vi "getSweepWaveforms.vi"(8 "error in (no error)":errorcluster, 11 "Instrument.LockinAPI in":refnum<class "Instrument.LockinAPI.lvclass">) -> (0 "error out":errorcluster, 1 "Sweep_AI":waveform(dbl)[](array[waveform]), 2 "Sweep_AO":waveform(dbl)[](array[waveform]), 3 "Instrument.LockinAPI out":refnum<class "Instrument.LockinAPI.lvclass">)   [LabVIEW 2019, in "Instrument.LockinAPI.lvclass"]
doc: "API to get the results of lockin calculation.\n\nIf address=\"\", this API reads from localhost\nIf address is remote lockin, you need to add this computer to allowed whitelist on the lockin computer you are trying to access."
uses:
  Instrument.LockinAPI.lvclass
  C:/Users/patrick/Documents/GitHub/Instrument-Framework/lvsrc/Instrument/Instrument.lvclass
  Typedefs/API/LockinAPI.Commands--Enum.ctl
  06e2ff75-1166-4892-8dfd-d8385005f928.vi
  06e2ff75-1166-4892-8dfd-d8385005f928.vi/f68ae031-2bc9-4b14-8172-68b8d1320710.vi
  06e2ff75-1166-4892-8dfd-d8385005f928.vi/f68ae031-2bc9-4b14-8172-68b8d1320710.vi/c120edc0-3eca-4408-adb5-28e9c0c7fff1.vi
  06e2ff75-1166-4892-8dfd-d8385005f928.vi/f68ae031-2bc9-4b14-8172-68b8d1320710.vi/c120edc0-3eca-4408-adb5-28e9c0c7fff1.vi/e50917fa-9e4a-4e04-9c38-a1a604490af2.vi
  06e2ff75-1166-4892-8dfd-d8385005f928.vi/f68ae031-2bc9-4b14-8172-68b8d1320710.vi/c120edc0-3eca-4408-adb5-28e9c0c7fff1.vi/56e2ec84-47dc-4db2-833f-128f254202da.vi
  Instrument/Protected/Validate API method.vi
  Instrument/Private/Get RC Connection Status.vi
  Instrument/API/Send and Receive.vi
  <vilib>/Utility/Data Type/Get Type Information.vi
  <vilib>/JDP Science/JSONtext/JSON text to Variant.vi
  <vilib>/JDP Science/JSONtext/LVClass Serializer/JSONtext LVClass Serializer.lvclass
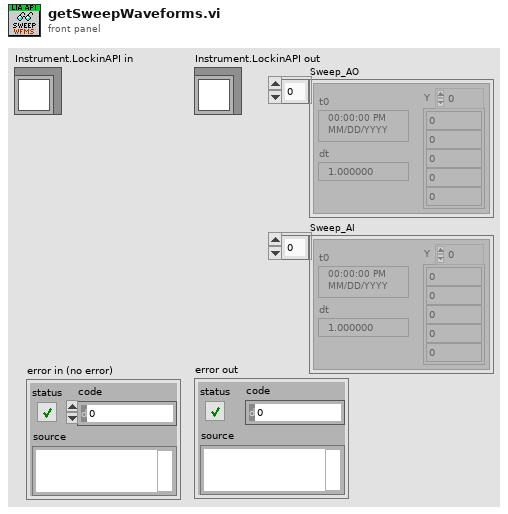
[diagram p1: front panel]
types:
  T1 = typedef "Instrument.LockinAPI.lvclass/LockinAPI.Commands--Enum.ctl" = enum16{"setAI", "setAO", "setAO_Amplitude", "setAO_DC", "setAO_Frequency", "setAO_Phase", "setAO_Function", "setAO_I+", "setREF", "setREF_Frequency", "setREF_Phase", "setREF_TC", "setREF_Roll-Off", "setDAQ", "setSampling", "setOffset", "setState", "getState", "getAO", "getAI", "getResults", "getSampling", "getAOconfig", "getREFconfig", "setInputGain", "setOutputGain", "getInputGain", "getOutputGain", "setSamplingMode", "getSamplingMode", "setSweep", "setSweepTime", "setSweepTable", "getStatus", "getSweepResults", "getSweepWaveforms", "startSweep", "stopSweep", "setAUX", "getAUX"}
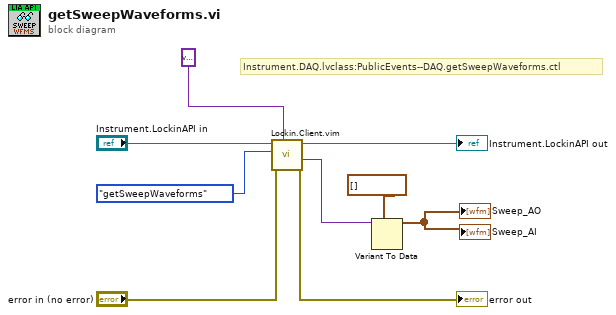
[diagram p0: block diagram]
diagram:
  # "Instrument.DAQ.lvclass:PublicEvents--DAQ.getSweepWaveforms.ctl"
  n1 = call "Lockin.Client.vim"("Data Out type"=variant, "error in (no error)"="error in (no error)", "Command"=LockinAPI.Commands--Enum."getSweepWaveforms", "Instrument.LockinAPI in"="Instrument.LockinAPI in") -> ("error out"=→"error out":errorcluster, "Data out"=w2:variant, "Instrument.LockinAPI out"=→"Instrument.LockinAPI out":refnum<class "Instrument.LockinAPI.lvclass">)  [unwired: 5 in]
  n2 = Variant To Data(type=waveform(dbl)[] [] ("X results"), Variant=w2) -> (data=→"Sweep_AO" →"Sweep_AI":waveform(dbl)[])  [unwired: 1 in, 1 out]
